vi "subVI_velocitymode_read_write_ADC_DAC.vi"(7 "ADC write":bool[](array[boolean])=[FALSE, FALSE, TRUE, FALSE, FALSE, TRUE, FALSE, FALSE, FALSE, FALSE, FALSE, FALSE, FALSE, FALSE, FALSE, FALSE], 8 "read only":bool, 9 "DAC":bool[](array[boolean])=[FALSE, FALSE, TRUE, FALSE, FALSE, TRUE, FALSE, FALSE, FALSE, FALSE, FALSE, FALSE, FALSE, FALSE, FALSE, FALSE], 10 "error in":errorcluster, 11 "FPGA VI Reference In":refnum<k20>) -> (0 "FPGA VI Reference Out":refnum<k20>, 1 "dec":u32, 2 "GAIN":i16, 3 "UNI":i16, 4 "error out":errorcluster)   [LabVIEW 2018]
uses:
  <vilib>/Utility/error.llb/Error Cluster From Error Code.vi
  <vilib>/rvi/errors/niLvFpgaAdjustHostInterfaceError.vi
  <vilib>/rvi/interface/nirviReadWriteControl/nirviReadWriteControl.xnode
  <vilib>/rvi/interface/Simulation/niFpgaSimulationCallBeginRW.vi
  NiFpgaLv.dll
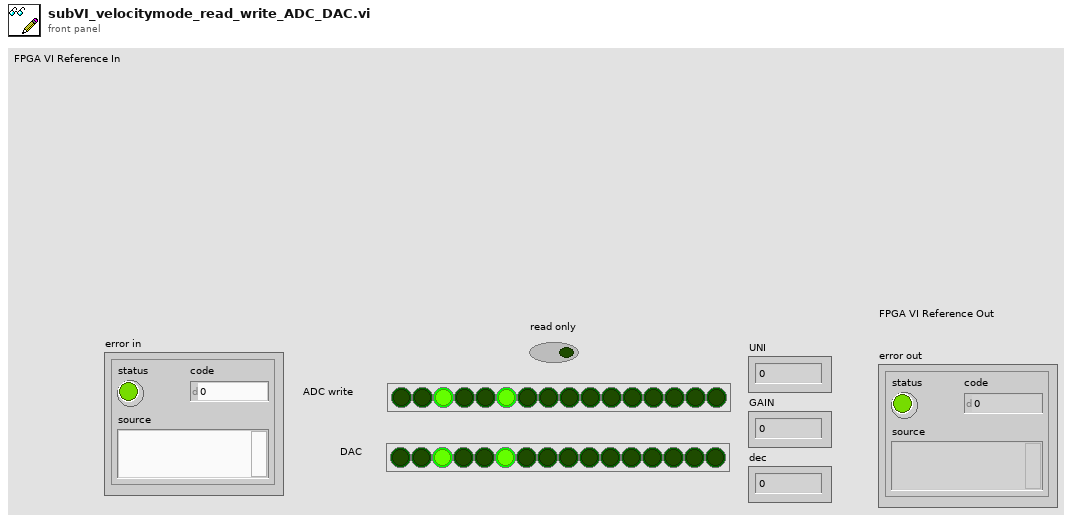
[diagram p1: front panel]
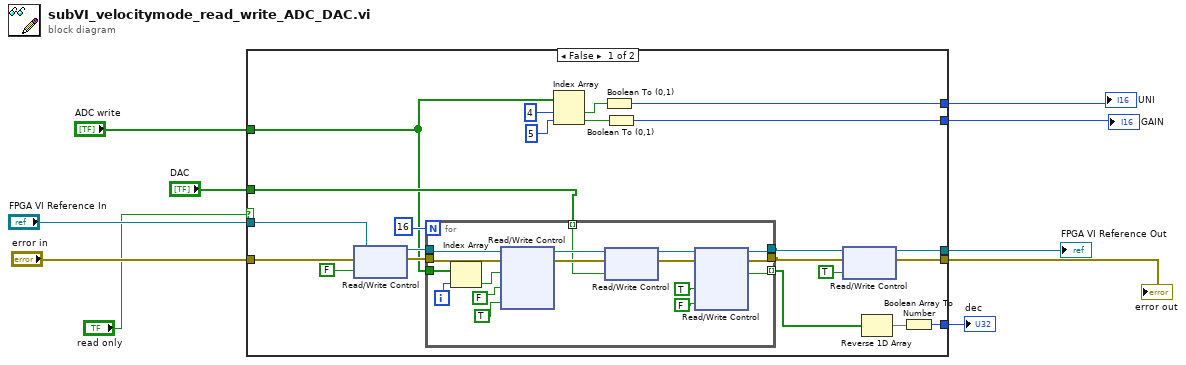
[diagram p0: block diagram]
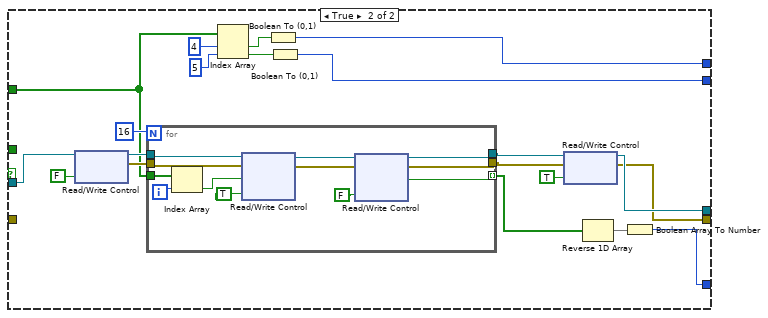
[diagram p2: hidden frame]
diagram:
  n1 = case shown="False" "read only" {
    tunnel: [w32 w54] -> w10
    tunnel: [w31 w53] -> w9
    tunnel: "DAC" -> [w21 _]
    tunnel: "error in" -> [w19 _]
    tunnel: [w18 w56] -> w7
    tunnel: [w17 w55] -> w6
    tunnel: "ADC write" -> [w16 w51]
    tunnel: [w15 w50] -> w4
    tunnel: "FPGA VI Reference In" -> [w12 w52]
    frame False {
      n2 = xnode "Read/Write Control"("FPGA VI Reference In"=w12, "error in"=w19, "CS"=FALSE) -> ("FPGA VI Reference Out"=w24:refnum<k20>, "error out"=w23:errorcluster)
      n3 = for {
        N: 16 -> [_]
        tunnel: w24 -> [w40]
        tunnel: w23 -> [w39]
        tunnel: [w35] -> w14 mode=indexing
        tunnel: [w34] -> w26
        tunnel: [w33] -> w25
        tunnel: w16 -> [w38]
        tunnel: w21 -> [w36] mode=indexing
        i -> [w37]
        n4 = Index Array(array=w38, index=w37) -> (element=w49:bool)
        n5 = xnode "Read/Write Control"("FPGA VI Reference In"=w40, "error in"=w39, "MOSI1"=w49, "CLK2"=FALSE ("CLK"), "CLK1"=TRUE ("CLK")) -> ("FPGA VI Reference Out"=w46:refnum<k20>, "error out"=w45:errorcluster)
        n6 = xnode "Read/Write Control"("FPGA VI Reference In"=w46, "error in"=w45, "MOSI2"=w36) -> ("FPGA VI Reference Out"=w44:refnum<k20>, "error out"=w43:errorcluster)
        n7 = xnode "Read/Write Control"("FPGA VI Reference In"=w44, "error in"=w43, "CLK2"=TRUE, "CLK1"=FALSE) -> ("FPGA VI Reference Out"=w34:refnum<k20>, "error out"=w33:errorcluster, "MISO1"=w35:bool)
      }
      n8 = Index Array(array=w16, index #1=4 ("index"), index #2=5 ("index")) -> (element #1=w28:bool, element #2=w27:bool)
      n9 = Boolean To (0,1)(Boolean=w28) -> (0, 1=w32:i16)
      n10 = Boolean To (0,1)(Boolean=w27) -> (0, 1=w31:i16)
      n11 = xnode "Read/Write Control"("FPGA VI Reference In"=w26, "error in"=w25, "CS"=TRUE) -> ("FPGA VI Reference Out"=w18:refnum<k20>, "error out"=w17:errorcluster)
      n12 = Reverse 1D Array(array=w14) -> (reversed array=w13:bool[])
      n13 = Boolean Array To Number(Boolean array=w13) -> (number=w15:u32)
    }
    frame True {
      n14 = xnode "Read/Write Control"("FPGA VI Reference In"=w52, "CS"=FALSE) -> ("FPGA VI Reference Out"=w66:refnum<k20>, "error out"=w67:errorcluster)  [unwired: 1 in]
      n15 = for {
        N: 16 -> [_]
        tunnel: w66 -> [w78]
        tunnel: w67 -> [w77]
        tunnel: [w74] -> w68 mode=indexing
        tunnel: [w73] -> w64
        tunnel: [w72] -> w65
        tunnel: w51 -> [w76]
        i -> [w75]
        n16 = Index Array(array=w76, index=w75) -> (element=w81:bool)
        n17 = xnode "Read/Write Control"("FPGA VI Reference In"=w78, "error in"=w77, "MOSI1"=w81, "CLK1"=TRUE ("CLK")) -> ("FPGA VI Reference Out"=w71:refnum<k20>, "error out"=w70:errorcluster)
        n18 = xnode "Read/Write Control"("FPGA VI Reference In"=w71, "error in"=w70, "CLK1"=FALSE ("CLK2")) -> ("FPGA VI Reference Out"=w73:refnum<k20>, "error out"=w72:errorcluster, "MISO1"=w74:bool)
      }
      n19 = Index Array(array=w51, index #1=4 ("index"), index #2=5 ("index")) -> (element #1=w62:bool, element #2=w63:bool)
      n20 = Boolean To (0,1)(Boolean=w62) -> (0, 1=w54:i16)
      n21 = Boolean To (0,1)(Boolean=w63) -> (0, 1=w53:i16)
      n22 = xnode "Read/Write Control"("FPGA VI Reference In"=w64, "error in"=w65, "CS"=TRUE) -> ("FPGA VI Reference Out"=w56:refnum<k20>, "error out"=w55:errorcluster)
      n23 = Reverse 1D Array(array=w68) -> (reversed array=w69:bool[])
      n24 = Boolean Array To Number(Boolean array=w69) -> (number=w50:u32)
    }
  }
  "UNI" <- w10
  "GAIN" <- w9
  "dec" <- w4
  "FPGA VI Reference Out" <- w7
  "error out" <- w6
